vi "APC_9056_TcoolantControl.vi"(1 "LoadIni?":bool, 2 "PC_ControlSettings":T1={"Spark advance [CADBTDC]"=0.0, "Pref"=0.0, "O2ref"=0.0, "DI advance [CADBTDC]"=0.0, "DI duration [ms] "=0.0, "CO2ref"=0.0, "PFI duration [ms]"=0.0, "IMEP ref"=0.0, "Speed ref"=0.0, "IGN enable"=TRUE, "DI enable"=TRUE, "CL PFI\n lambda"=TRUE, "CL PFI\nIMEP"=FALSE, "Activate\ncylinder"=[FALSE, FALSE, FALSE, FALSE, FALSE, FALSE], "Force idling"=FALSE, "Force motoring"=FALSE, "ETP resync"=FALSE, "Requested mode"=0, "Clear Sync Errors"=FALSE, "toggle TDC"=FALSE, "l ref"=0.0, "PID control references"={"NG"=FALSE, "Ar"=FALSE, "O2"=FALSE, "Intake vent"=FALSE, "Cross vent"=FALSE, "Exhaust vent"=FALSE, "NG control mode"=0, "NG-FC-001-REF"=0.0, "WF-OA-002-REF"=0.0, "IMEP-REF"=0.0, "Nm-REF"=0.0, "Ar control mode"=0, "AR-PC-002-REF"=0.0, "WF-PT-004-REF"=0.0, "O2 control mode"=0, "O2-FC-001-REF"=0.0, "WF-OA-001-REF"=0.0, "Tcoolant control  mode"=0, "EC-FC-001-REF"=0.0, "EC-TT-001-REF"=0.0, "Texh control mode"=0, "SW-FC-004-REF"=0.0, "SW-FT-002-REF"=0.0, "WF-TT-004-REF"=0.0, "Toil control mode"=0, "SW-FC-009-REF"=0.0, "SW-FT-004-REF"=0.0, "EO-TT-001-REF"=0.0, "AIC201_CO2_ConcTarget"=0.0, "O2_FF_NG"=FALSE, "Dyno control mode"=0, "Membrane control mode"=0, "AR-FT-001-REF"=0.0, "MTR modbus floats"=[0.0, 0.0, 0.0, 0.0, 0.0, 0.0, 0.0, 0.0, 0.0, 0.0, 0.0, 0.0, 0.0, 0.0, 0.0, 0.0, 0.0, 0.0, 0.0], "MTR modbus u16"=[0, 0, 0, 0, 0, 0, 0], "MTR HB"=FALSE, "PC_HB"=FALSE, "EMERGENCY STOP"=FALSE}, "CA50setpoint [CADATDC]"=0.0, "CA50 control"=TRUE, "Knock control"=TRUE, "CLEAR EMERGENCY STOP"=FALSE, "EMERGENCY STOP"=FALSE}, 3 "input cluster":T3) -> (0 "EC-FC-001-REF":dbl format="%.2f")   [LabVIEW 2020]
uses:
  controls/APC_PIDCluster.ctl
  controls/APC_ControlSettings.ctl
  controls/APC_PIDcontrolSettings.ctl
  controls/APC_cascadePIDsettings.ctl
  <vilib>/addons/control/pid/pid.llb/PID Advanced (DBL).vi
  <vilib>/Utility/xml.llb/Read From XML File(string).vi
  <vilib>/Utility/xml.llb/Write to XML File(string).vi
  <vilib>/addons/control/pid/NI_PID_pid.lvlib
panel:
  out "direct?":bool
  out "Direct control":dbl format="%.2f"
  in  "EC-FC-001-REF (manual)":dbl
  in  "save":bool
  in  "load":bool
  out "Tcoolant control mode":u8
  out "EC-TT-001":dbl=2293.506542256783
  in  "FF control":dbl format="%.2f"
  in  "reinitialize? (F)":bool
  in  "EC-TT-001-REF (manual)":dbl
  in  "Tcoolant control mode (manual)":u8
  in  "PID gains":T4={"proportional gain (Kc)"=1.0, "integral time (Ti, min)"=0.01, "derivative time (Td, min)"=0.0} {"derivative time (Td, min)" format="%.3f"; "integral time (Ti, min)" format="%.3f"; "proportional gain (Kc)" format="%.3f"}
  in  "PID setpoint range":cluster{"setpoint high":dbl, "setpoint low":dbl}={"setpoint high"=100.0, "setpoint low"=0.0} {"setpoint high" format="%.2f"; "setpoint low" format="%.2f"}
  in  "PID output range":cluster{"output high":dbl, "output low":dbl}={"output high"=100.0, "output low"=-100.0} {"output low" format="%.2f"; "output high" format="%.2f"}
  in  "Override PC PID references":bool
  in  "Safe mode control":dbl format="%.2f"
  in  "learn?":bool
  out "CL on?":bool
  out "setpoint":dbl format="%.2f"
  # "Tcoolant control"
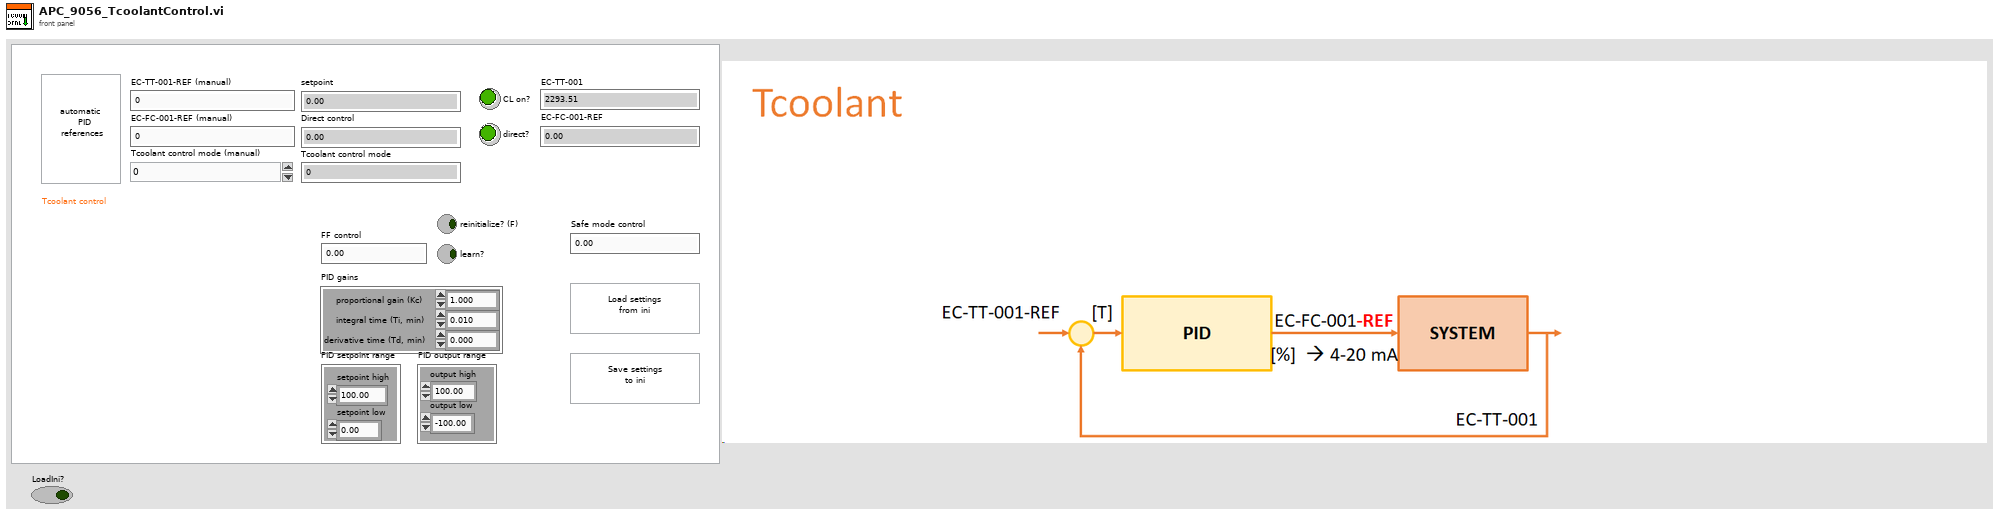
[diagram p1: front panel]
types:
  T1 = typedef "APC_ControlSettings.ctl" = cluster{"Spark advance [CADBTDC]":dbl, "Pref":dbl, "O2ref":dbl, "DI advance [CADBTDC]":dbl, "DI duration [ms] ":dbl, "CO2ref":dbl, "PFI duration [ms]":dbl, "IMEP ref":dbl, "Speed ref":dbl, "IGN enable":bool, "DI enable":bool, "CL PFI\n lambda":bool, "CL PFI\nIMEP":bool, "Activate\ncylinder":bool[], "Force idling":bool, "Force motoring":bool, "ETP resync":bool, "Requested mode":i8, "Clear Sync Errors":bool, "toggle TDC":bool, "l ref":dbl, "PID control references":T2, "CA50setpoint [CADATDC]":dbl, "CA50 control":bool, "Knock control":bool, "CLEAR EMERGENCY STOP":bool, "EMERGENCY STOP":bool}
  T2 = typedef "APC_PIDcontrolSettings.ctl" = cluster{"NG":bool, "Ar":bool, "O2":bool, "Intake vent":bool, "Cross vent":bool, "Exhaust vent":bool, "NG control mode":u8, "NG-FC-001-REF":dbl, "WF-OA-002-REF":dbl, "IMEP-REF":dbl, "Nm-REF":dbl, "Ar control mode":u8, "AR-PC-002-REF":dbl, "WF-PT-004-REF":dbl, "O2 control mode":u8, "O2-FC-001-REF":dbl, "WF-OA-001-REF":dbl, "Tcoolant control  mode":u8, "EC-FC-001-REF":dbl, "EC-TT-001-REF":dbl, "Texh control mode":u8, "SW-FC-004-REF":dbl, "SW-FT-002-REF":dbl, "WF-TT-004-REF":dbl, "Toil control mode":u8, "SW-FC-009-REF":dbl, "SW-FT-004-REF":dbl, "EO-TT-001-REF":dbl, "AIC201_CO2_ConcTarget":dbl, "O2_FF_NG":bool, "Dyno control mode":u8, "Membrane control mode":u8, "AR-FT-001-REF":dbl, "MTR modbus floats":sgl[], "MTR modbus u16":u16[], "MTR HB":bool, "PC_HB":bool, "EMERGENCY STOP":bool}
  T3 = typedef "APC_PIDCluster.ctl" = cluster{"AR-FT-001":dbl, "O2-FC-001":dbl, "SW-FT-004":dbl, "SW-FT-002":dbl, "WF-OA-002":dbl, "WF-PT-004":dbl, "WF-OA-001":dbl, "EC-TT-001":dbl, "WF-TT-004":dbl, "EC-FC-001":dbl, "NG-FC-001":dbl, "EO-TT-001":dbl, "SW-FC-008":dbl, "SW-FC-004":dbl, "IMEPn6":dbl, "TORQUE":dbl, "CylPresWarnings":dbl, "CylPresErrors":dbl, "NG-FT-001":dbl, "EngineSpeed_rpm":dbl}
  T4 = cluster{"proportional gain (Kc)":dbl, "integral time (Ti, min)":dbl, "derivative time (Td, min)":dbl}
  T5 = typedef "APC_cascadePIDsettings.ctl" = cluster{"HL FF control":dbl, "LL FF control":dbl, "HL PID gains":cluster{"proportional gain (Kc)":dbl, "integral time (Ti, min)":dbl, "derivative time (Td, min)":dbl}, "LL PID gains":cluster{"proportional gain (Kc)":dbl, "integral time (Ti, min)":dbl, "derivative time (Td, min)":dbl}, "HL PID setpoint range":cluster{"setpoint high":dbl, "setpoint low":dbl}, "HL PID output range":cluster{"output high":dbl, "output low":dbl}, "LL PID setpoint range":cluster{"setpoint high":dbl, "setpoint low":dbl}, "LL PID output range":cluster{"output high":dbl, "output low":dbl}, "Safe mode control":dbl}
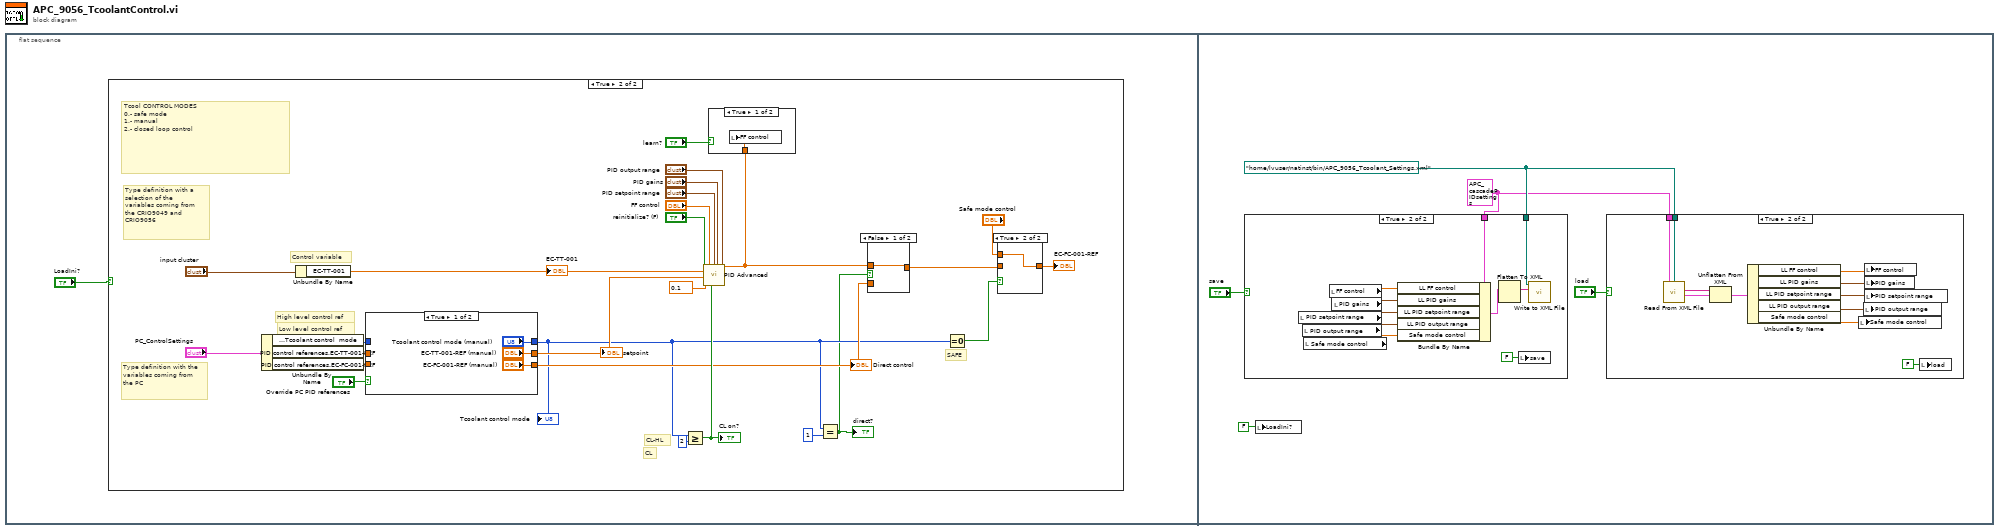
[diagram p0: block diagram]
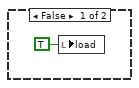
[diagram p2: hidden frame]
diagram:
  n1 = flat-sequence {
    frame #0 {
      n2 = case shown="True" "LoadIni?" {
        frame False {
          n3 = local write "load"(TRUE ("load")) -> ()
        }
        frame True {
          # "Type definition with a selection of the variables coming from the CRIO9049 and CRIO9056"
          # "Type definition with the variables coming from the PC"
          # "Low level control ref"
          # "High level control ref"
          # "Control variable"
          # "SAFE"
          # "CL-HL"
          # "CL"
          # "Tcool CONTROL MODES\n0.- safe mode\n1.- manual\n2.- closed loop control"
          n4 = Unbundle By Name("PC_ControlSettings") -> ("PID control references.Tcoolant control  mode"=w16:u8, "PID control references.EC-TT-001-REF"=w15:dbl, "PID control references.EC-FC-001-REF"=w9:dbl)
          n5 = Unbundle By Name("input cluster") -> ("EC-TT-001"=w13:dbl)
          "EC-TT-001" <- w13
          n6 = case shown="True" "Override PC PID references" {
            tunnel: w16 -> [_ w39]
            tunnel: w15 -> [_ w38]
            tunnel: ["Tcoolant control mode (manual)" w39] -> w4
            tunnel: ["EC-TT-001-REF (manual)" w38] -> w10
            tunnel: ["EC-FC-001-REF (manual)" w37] -> w5
            tunnel: w9 -> [_ w37]
            frame True {
            }
            frame False {
            }
          }
          "setpoint" <- w10
          "Tcoolant control mode" <- w4
          "Direct control" <- w5
          n7 = Greater Or Equal?(x=w4, y=u8 2) -> (x >= y?=w26:bool)
          "CL on?" <- w26
          n8 = call-poly <vilib>:"PID Advanced.vi"("setpoint"=w10, "output range"="PID output range", "auto? (T)"=w26, "manual control"="FF control", "process variable"=w13, "setpoint range"="PID setpoint range", "PID gains"="PID gains", "dt (s)"=0.1, "reinitialize? (F)"="reinitialize? (F)") -> ("output"=w6:dbl)  [unwired: 5 in, 1 out]
          n9 = case shown="True" "learn?" {
            tunnel: w6 -> [w31 _]
            frame True {
              n10 = local write "FF control"(w31) -> ()
            }
            frame False {
            }
          }
          n11 = Equal?(x=w4, y=u8 1) -> (x = y?=w3:bool)
          "direct?" <- w3
          n12 = case shown="False" w3 {
            tunnel: [w29 w30] -> w7
            tunnel: w6 -> [w29 _]
            tunnel: w5 -> [_ w30]
            frame False {
            }
            frame True {
            }
          }
          n13 = Equal To 0?(x=w4) -> (x = 0?=w28:bool)
          n14 = case shown="True" w28 {
            tunnel: [w32 w33] -> w22
            tunnel: "Safe mode control" -> [_ w33]
            tunnel: w7 -> [w32 _]
            frame False {
            }
            frame True {
            }
          }
          "EC-FC-001-REF" <- w22
        }
      }
    }
    frame #1 {
      w42 = path "/home/lvuser/natinst/bin/APC_9056_Tcoolant_Settings.xml" ("XML File Path")
      w41 = T5 {"HL FF control"=0.0, "LL FF control"=0.0, "HL PID gains"={"proportional gain (Kc)"=1.0, "integral time (Ti, min)"=0.01, "derivative time (Td, min)"=0.0}, "LL PID gains"={"proportional gain (Kc)"=1.0, "integral time (Ti, min)"=0.01, "derivative time (Td, min)"=0.0}, "HL PID setpoint range"={"setpoint high"=100.0, "setpoint low"=0.0}, "HL PID output range"={"output high"=0.0, "output low"=0.0}, "LL PID setpoint range"={"setpoint high"=100.0, "setpoint low"=0.0}, "LL PID output range"={"output high"=10.0, "output low"=-10.0}, "Safe mode control"=0.0} ("Cluster")
      n15 = case shown="True" "save" {
        tunnel: w42 -> [_ w57]
        tunnel: w41 -> [_ w56]
        frame False {
        }
        frame True {
          n16 = local read "PID setpoint range"() -> (w62:cluster{"setpoint high":dbl, "setpoint low":dbl})
          n17 = local read "PID output range"() -> (w61:cluster{"output high":dbl, "output low":dbl})
          n18 = local read "Safe mode control"() -> (w60:dbl)
          n19 = local read "FF control"() -> (w64:dbl)
          n20 = local read "PID gains"() -> (w63:T4)
          n21 = Bundle By Name(cluster=w56, "LL FF control"=w64, "LL PID gains"=w63, "LL PID setpoint range"=w62, "LL PID output range"=w61, "Safe mode control"=w60) -> (w59:T5)
          n22 = Flatten To XML(6:w59) -> (2:w58:string)
          n23 = local write "save"(FALSE ("load")) -> ()
          n24 = call-poly <vilib>:"Write to XML File.vi"("XML Input"=w58, "XML File Path"=w57) -> ()  [unwired: 7 in, 3 out]
        }
      }
      n25 = local write "LoadIni?"(FALSE ("LoadIni?")) -> ()
      n26 = case shown="True" "load" {
        tunnel: w42 -> [_ w53]
        tunnel: w41 -> [_ w52]
        frame False {
        }
        frame True {
          n27 = call-poly <vilib>:"Read From XML File.vi"("XML File Path"=w53) -> ("XML Elements"=w54:string)  [unwired: 8 in, 2 out]
          n28 = Unflatten From XML(xml string=w54, type=w52) -> (value=w51:T5)  [unwired: 1 in, 1 out]
          n29 = Unbundle By Name(w51) -> ("LL FF control"=w50:dbl, "LL PID gains"=w49:T4, "LL PID setpoint range"=w48:cluster{"setpoint high":dbl, "setpoint low":dbl}, "LL PID output range"=w47:cluster{"output high":dbl, "output low":dbl}, "Safe mode control"=w46:dbl)
          n30 = local write "Safe mode control"(w46) -> ()
          n31 = local write "PID output range"(w47) -> ()
          n32 = local write "FF control"(w50) -> ()
          n33 = local write "PID gains"(w49) -> ()
          n34 = local write "PID setpoint range"(w48) -> ()
          n35 = local write "load"(FALSE ("save")) -> ()
        }
      }
    }
  }
